vi "WPI_DMAOpenExternal.vi"(6 "Divisor":u32=1, 8 "error in (no error)":errorcluster, 9 "Host Buffer Depth (Samples)":u32=512, 10 "ExternalSampleClocks":T5(array[cluster])) -> (0 "error out":errorcluster, 3 "DMARef":T6)   [LabVIEW 2017]
doc: "Opens a reference to the DMA stream from the FPGA of the roboRIO. You must open a reference before using any other VIs on this palette. You can have only one DMA stream open at a time. If you want to open a new DMA stream, use the Close VI to close the reference to the current DMA stream first.\n\nUses an external sample clock to specify the frequency at which the FPGA sends data samples to the host buffer. Use this VI to specify the digital input or analog trigger output that causes the FPGA on the roboRIO to transfer data to the host buffer.\n\nThis software is licensed. Open the labview\\readme\\WPI Robotics Library Open Source License.txt file for more information."
uses:
  <vilib>/Rock Robotics/WPI/DMA/WPI_DMARef.ctl
  <vilib>/Rock Robotics/SystemInterfaces/CounterEncoderSourceConvertion/FPGA_CounterEncoderSourceConvertionLVSourceType.ctl
  <vilib>/Rock Robotics/SystemInterfaces/DIO/FPGA_DIODigitalSourceChannel.ctl
  <vilib>/Rock Robotics/SystemInterfaces/AnalogTrigger/FPGA_AnalogTriggerIndex.ctl
  <vilib>/Rock Robotics/SystemInterfaces/AnalogTrigger/FPGA_AnalogTriggerOutType.ctl
  <vilib>/Rock Robotics/SystemInterfaces/DMA/FPGA_DMAWriteConfigOperation.ctl
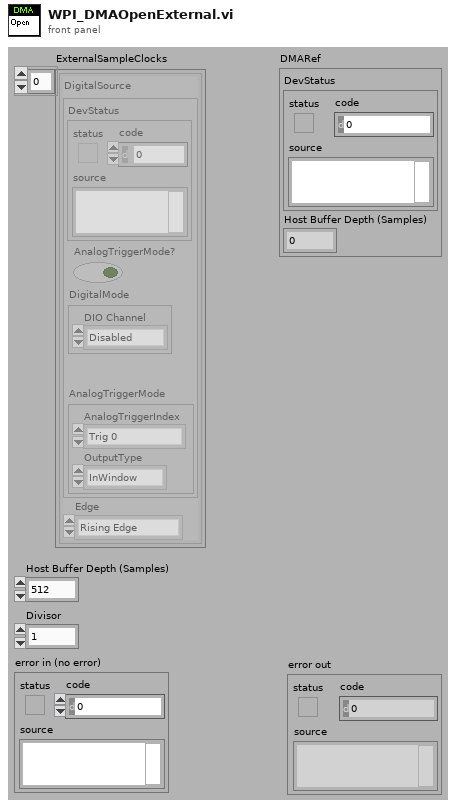
[diagram p1: front panel]
types:
  T1 = typedef "FPGA_CounterEncoderSourceConvertionLVSourceType.ctl" = cluster{"DevStatus":errorcluster, "AnalogTriggerMode?":bool, "DigitalMode":cluster{"DIO Channel":T2}, "AnalogTriggerMode":cluster{"AnalogTriggerIndex":T3, "OutputType":T4}}
  T2 = typedef "FPGA_DIODigitalSourceChannel.ctl" = enum8{"DIO 0", "DIO 1", "DIO 2", "DIO 3", "DIO 4", "DIO 5", "DIO 6", "DIO 7", "DIO 8", "DIO 9", "DIO MXP 0", "DIO MXP 1", "DIO MXP 2", "DIO MXP 3", "DIO MXP 4", "DIO MXP 5", "DIO MXP 6", "DIO MXP 7", "DIO MXP 8", "DIO MXP 9", "DIO MXP 10", "DIO MXP 11", "DIO MXP 12", "DIO MXP 13", "DIO MXP 14", "DIO MXP 15", "Disabled"}
  T3 = typedef "FPGA_AnalogTriggerIndex.ctl" = enum8{"Trig 0", "Trig 1", "Trig 2", "Trig 3", "Trig 4", "Trig 5", "Trig 6", "Trig 7", "Invalid"}
  T4 = typedef "FPGA_AnalogTriggerOutType.ctl" = enum16{"InWindow", "TriggerState", "Rising", "Falling"}
  T5 = cluster{"DigitalSource":T1, "Edge":enum16{"Rising Edge", "Falling Edge", "Raising & Falling Edge", "Disabled"}}[]
  T6 = typedef "WPI_DMARef.ctl" = cluster{"DevStatus":errorcluster, "Host Buffer Depth (Samples)":u32}
  T7 = cluster{"DigitalSource":T1, "RisingEdge":bool, "FallingEdge":bool}
  T8 = cluster{"ExternalClock":bool, "ExternalTriggers":cluster{"DigitalSource":T1, "RisingEdge":bool, "FallingEdge":bool}[]}
  T9 = typedef "FPGA_DMAWriteConfigOperation.ctl" = enum16{"Update Pause", "Update Enable", "Update SampleClock"}
  T10 = typedef "WPI_DMAChannelTypeEnum.ctl" = enum16{"AI (Raw)", "AI (Avg)", "Accumulator", "DI (Raw) Onboard", "DI (Filtered) Onboard", "DI (Raw) MXP", "DI (Filtered) MXP", "Analog Trigger", "Counter", "Counter (Timer)", "Encoder", "Encoder (Timer)", "Time Stamp"}
  T11 = cluster{"Channel Type":T10, "Channel Number":u8}[]
  T12 = enum16{"Rising Edge", "Falling Edge", "Raising & Falling Edge", "Disabled"}
  T13 = typedef "FPGA_DMADevRef.ctl" = cluster{"DevStatus":errorcluster}
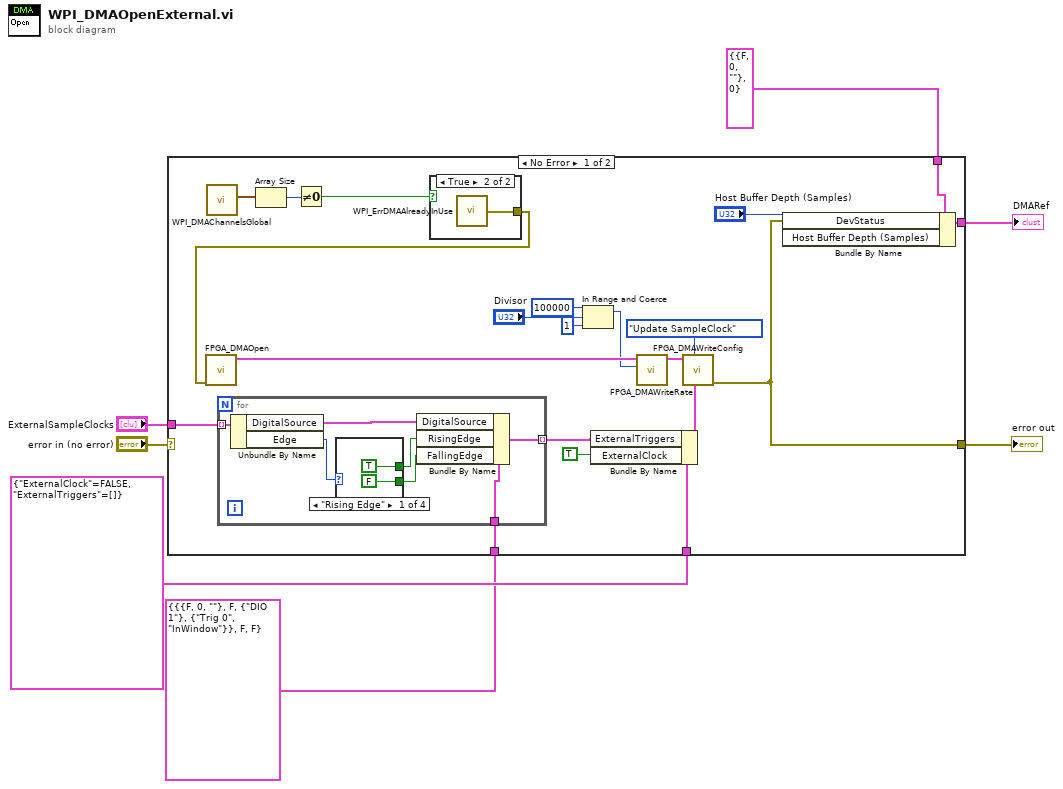
[diagram p0: block diagram]
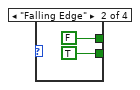
[diagram p2: hidden frame]
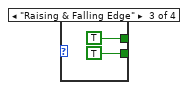
[diagram p3: hidden frame]
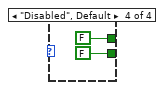
[diagram p4: hidden frame]
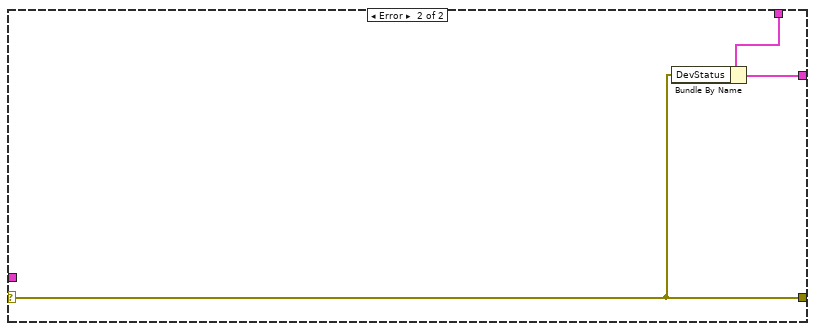
[diagram p6: hidden frame]
diagram:
  n1 = case shown="No Error" "error in (no error)" {
    selector: "error in (no error)" -> [_ w46]
    tunnel: [w19 w46] -> w6
    tunnel: [w27 w47] -> w5
    tunnel: T6 {"DevStatus"={"status"=FALSE, "code"=0, "source"=""}, "Host Buffer Depth (Samples)"=0} ("DMARef") -> [w28 w45]
    tunnel: T8 {"ExternalClock"=FALSE, "ExternalTriggers"=[]} ("SampleClock") -> [w21 _]
    tunnel: "ExternalSampleClocks" -> [w10 _]
    tunnel: T7 {"DigitalSource"={"DevStatus"={"status"=FALSE, "code"=0, "source"=""}, "AnalogTriggerMode?"=FALSE, "DigitalMode"={"DIO Channel"=enum."DIO 1"}, "AnalogTriggerMode"={"AnalogTriggerIndex"=enum."Trig 0", "OutputType"=enum."InWindow"}}, "RisingEdge"=FALSE, "FallingEdge"=FALSE} -> [w9 _]
    frame No Error {
      n2 = call <vilib>:"WPI_DMAChannelsGlobal.vi"() -> ("Channels Out"=w26:T11)  [unwired: 4 in, 7 out]
      n3 = for {
        tunnel: w10 -> [w35] mode=indexing
        tunnel: w9 -> [w34]
        tunnel: [w29] -> w8 mode=indexing
        n4 = Unbundle By Name(w35) -> ("DigitalSource"=w32:T1, "Edge"=w33:T12)
        n5 = case shown="\"Rising Edge\"" w33 {
          tunnel: [TRUE FALSE TRUE FALSE] -> w31
          tunnel: [FALSE TRUE TRUE FALSE] -> w30
          frame "Rising Edge" {
          }
          frame "Falling Edge" {
          }
          frame "Raising & Falling Edge" {
          }
          frame "Disabled", Default {
          }
        }
        n6 = Bundle By Name(cluster=w34, "DigitalSource"=w32, "RisingEdge"=w31, "FallingEdge"=w30) -> (w29:T7)
      }
      n7 = Array Size(array=w26) -> (size(s)=w25:i32)
      n8 = Not Equal To 0?(x=w25) -> (x != 0?=w24:bool)
      n9 = case shown="True" w24 {
        tunnel: [_ w44] -> w23
        frame False {
        }
        frame True {
          n10 = call <vilib>:"WPI_ErrDMAAlreadyInUse.vi"() -> ("error out"=w44:errorcluster)
        }
      }
      n11 = call <vilib>:"FPGA_DMAOpen.vi"("error in (no error)"=w23) -> ("DMADevRef"=w17:T13)  [unwired: 10 out]
      n12 = In Range and Coerce(upper limit=u32 100000, x="Divisor", lower limit=u32 1) -> (coerced(x)=w12:u32)  [unwired: 1 out]
      n13 = Bundle By Name(cluster=w21, "ExternalTriggers"=w8, "ExternalClock"=TRUE) -> (w11:T8)
      n14 = call <vilib>:"FPGA_DMAWriteRate.vi"("Rate"=w12, "DMADevRef In"=w17) -> ("DMADevRef Out"=w16:T13)  [unwired: 1 in, 8 out]
      n15 = call <vilib>:"FPGA_DMAWriteConfig.vi"("SampleClock"=w11, "Operation"=FPGA_DMAWriteConfigOperation."Update SampleClock", "DMADevRef"=w16) -> ("error out"=w19:errorcluster)  [unwired: 3 in, 5 out]
      n16 = Bundle By Name(cluster=w28, "DevStatus"=w19, "Host Buffer Depth (Samples)"="Host Buffer Depth (Samples)") -> (w27:T6)
    }
    frame Error {
      n17 = Bundle By Name(cluster=w45, "DevStatus"=w46) -> (w47:T6)
    }
  }
  "error out" <- w6
  "DMARef" <- w5
